vi "Read U8 Array FIFO.vi"(7 "Channel Index":i32, 8 "error in (no error)":errorcluster, 9 "Timeout (ms)":i32, 11 "CIFCorePlugin in":refnum<class "CIFCorePlugin.lvclass">) -> (0 "error out":errorcluster, 1 "timed out?":bool, 2 "Data":u8[](array[numeric]) format="%.0x", 3 "CIFCorePlugin out":refnum<class "CIFCorePlugin.lvclass">, 4 "Header":T1)   [LabVIEW 2021, in "CIFCorePlugin.lvclass"]
uses:
  CIFCorePlugin.lvclass
  <vilib>/CIF Foundation/CIF Channels Core/ChannelCommon/typedef/FIFO Header.ctl
  CIFCorePlugin.lvclass/CIFCorePlugin.ctl
  <vilib>/CIF Foundation/CIF Channels Core/CIFChannels/CIFChannels.lvclass
  <vilib>/CIF Foundation/CIF Channels Core/ChannelCommon/ChannelCommon.lvlib
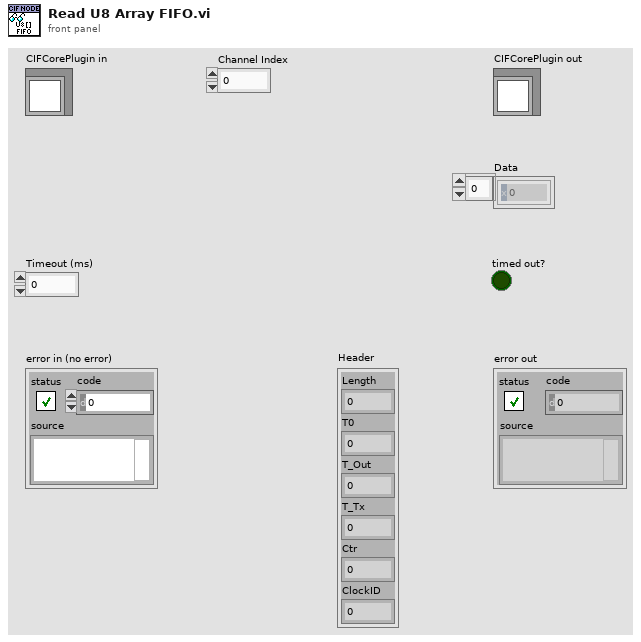
[diagram p1: front panel]
types:
  T1 = typedef "ChannelCommon.lvlib/FIFO Header.ctl" = cluster{"Length":u64, "T0":i64, "T_Out":i64, "T_Tx":i64, "Ctr":u64, "ClockID":u8}
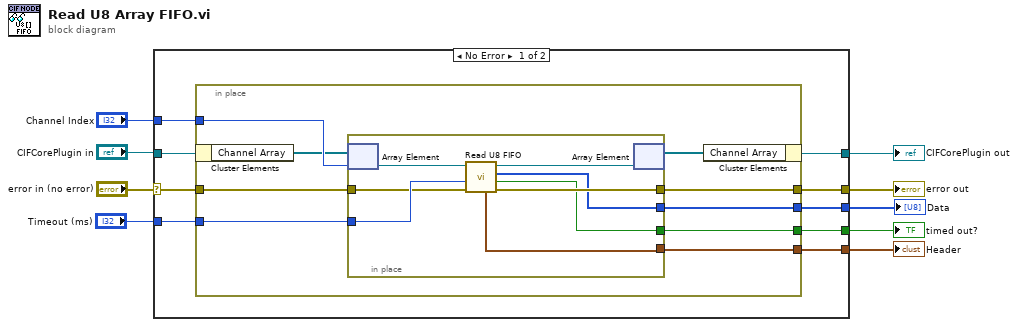
[diagram p0: block diagram]
diagram:
  n1 = case shown="No Error" "error in (no error)" {
    selector: "error in (no error)" -> [w18 w37]
    tunnel: [w17 w37] -> w7
    tunnel: [w14 w36] -> w8
    tunnel: "CIFCorePlugin in" -> [w15 w36]
    tunnel: [w16 _] -> w1
    tunnel: "Channel Index" -> [w13 _]
    tunnel: "Timeout (ms)" -> [w12 _]
    tunnel: [w11 _] -> w3
    tunnel: [w10 _] -> w2
    frame No Error {
      n2 = in-place {
        in-place-border: w18 -> [w19]
        in-place-border: [w20] -> w17
        in-place-border: [w27] -> w16
        in-place-border: w13 -> [w26]
        in-place-border: w12 -> [w25]
        in-place-border: [w24] -> w11
        in-place-border: [w23] -> w10
        n3 = in-place-cluster #1(w15) -> ("Channel Array"=w22:refnum<class "CIFChannels.lvclass">[])
        n4 = in-place {
          in-place-border: w19 -> [w33]
          in-place-border: [w31] -> w20
          in-place-border: [w29] -> w27
          in-place-border: w25 -> [w34]
          in-place-border: [w30] -> w24
          in-place-border: [w32] -> w23
          n5 = in-place-array #2(w22, w26) -> (w35:refnum<class "CIFChannels.lvclass">)
          n6 = call-dynamic "Read U8 FIFO.vi"("error in (no error)"=w33, "Timeout (ms)"=w34, "CIFChannels in"=w35) -> ("error out"=w31:errorcluster, "timed out?"=w30:bool, "Data out"=w29:u8[], "CIFChannels out"=w28:refnum<class "CIFChannels.lvclass">, "Header"=w32:T1)  [unwired: 4 in]
          n7 = in-place-array #2(w28) -> (w21:refnum<class "CIFChannels.lvclass">[])  [unwired: 1 out]
        }
        n8 = in-place-cluster #1("Channel Array"=w21) -> (w14:refnum<class "CIFCorePlugin.lvclass">)
      }
    }
    frame Error {
    }
  }
  "error out" <- w7
  "CIFCorePlugin out" <- w8
  "timed out?" <- w3
  "Header" <- w2
  "Data" <- w1
